vi "Check IP Config.vi"(7 "Retry wait time [ms]":u32=2000, 8 "Error In":errorcluster, 10 "TCP Configuration":T5, 11 "LINX Resource":T1) -> (0 "error out":errorcluster, 2 "TCP Config out":T5, 3 "LINX Resource Out":T1)   [LabVIEW 2019, in "LINXx.lvlib"]
uses:
  LINXx.lvlib
  <vilib>/MakerHub/LINX/Private/Device/Type Defs/TCP Config.ctl
  <vilib>/MakerHub/LINX/Private/Type Defs/LINX Ref.ctl
  <vilib>/MakerHub/LINX/Private/Type Defs/Platform.ctl
  <vilib>/MakerHub/LINX/Private/Type Defs/Interface.ctl
  <vilib>/MakerHub/LINX/Private/Device/Type Defs/LINX Device Config.ctl
  <vilib>/MakerHub/LINX/Private/Device/Type Defs/Channels.ctl
  <vilib>/Utility/error.llb/DialogType.ctl
  Public/Reset Target.ctl
  <vilib>/Utility/error.llb/Error Cluster From Error Code.vi
  <vilib>/ErrorRing/Error Ring.xnode
  <vilib>/MakerHub/LINX/Private/Device/Device.lvlib
  <vilib>/MakerHub/LINX/LMH-LINX.lvlib
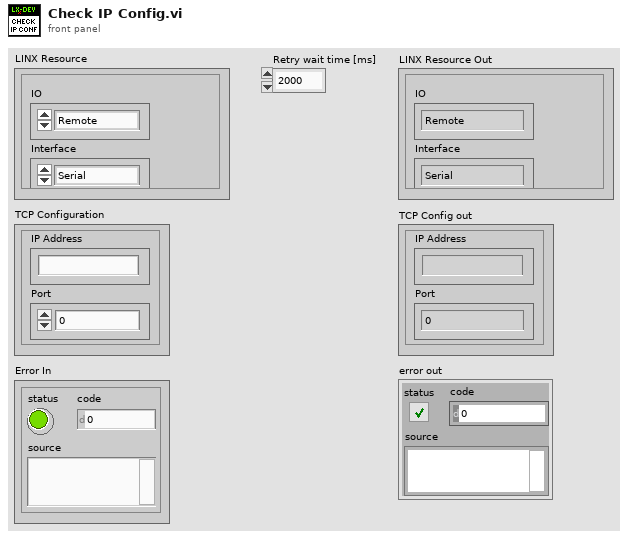
[diagram p1: front panel]
types:
  T1 = typedef "LMH-LINX.lvlib/LINX Ref.ctl" = cluster{"IO":T2, "Interface":T3, "LINX Device Config":T4}
  T2 = typedef "LMH-LINX.lvlib/Platform.ctl" = enum16{"Remote", "Local"}
  T3 = typedef "LMH-LINX.lvlib/Interface.ctl" = enum16{"Serial", "TCP"}
  T4 = typedef "LMH-LINX.lvlib/Device.lvlib/LINX Device Config.ctl" = cluster{"Interface":T3, "COM Port":refnum<visa-resource-name>, "TCP Configuration":T5, "Device Family":u8, "Device ID":u8, "Device Name":string, "TCP Ref":refnum<k5>, "Channels":T6}
  T5 = typedef "LMH-LINX.lvlib/Device.lvlib/TCP Config.ctl" = cluster{"IP Address":string, "Port":u16}
  T6 = typedef "LMH-LINX.lvlib/Channels.ctl" = cluster{"DI":u8[], "DO":u8[], "AI":u8[], "AO":u8[], "PWM":u8[], "QE":u8[], "UART":u8[], "I2C 2":u8[], "SPI":u8[], "CAN":u8[], "Servo":u8[], "AI Ref (V)":dbl, "AI Resolution (Bits)":u8, "AO Ref (V)":dbl, "AO Resolution (Bits)":u8}
  T7 = typedef "DialogType.ctl" = u16
  T8 = typedef "LINXx.lvlib/Reset Target.ctl" = enum16{"None", "Serial", "TCP", "Board"}
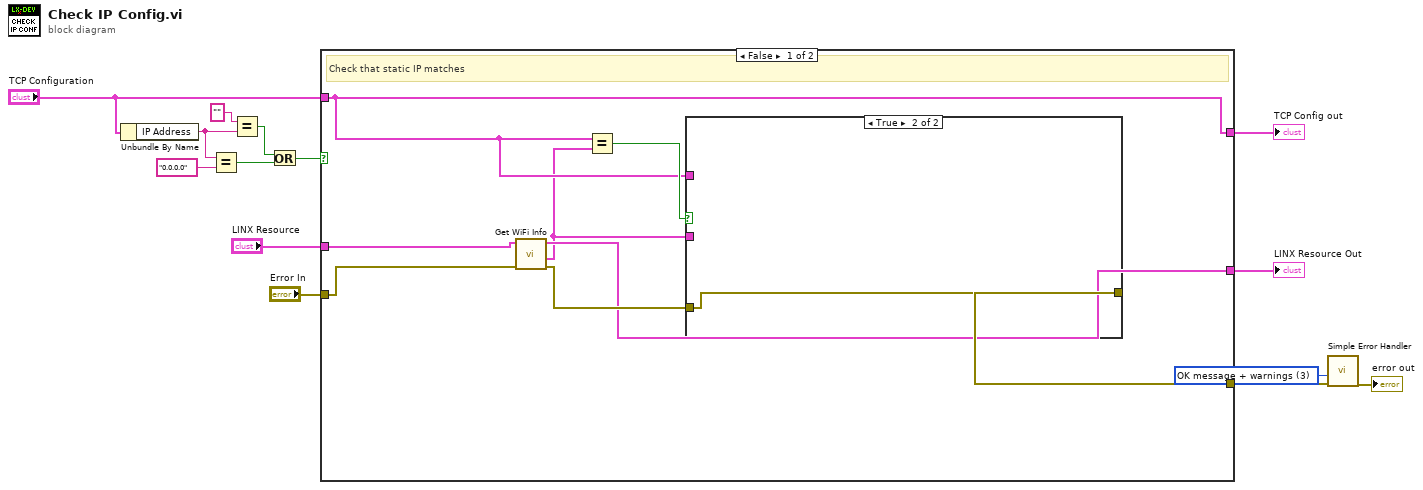
[diagram p0: block diagram]
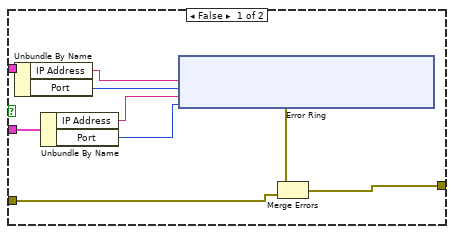
[diagram p2: hidden frame]
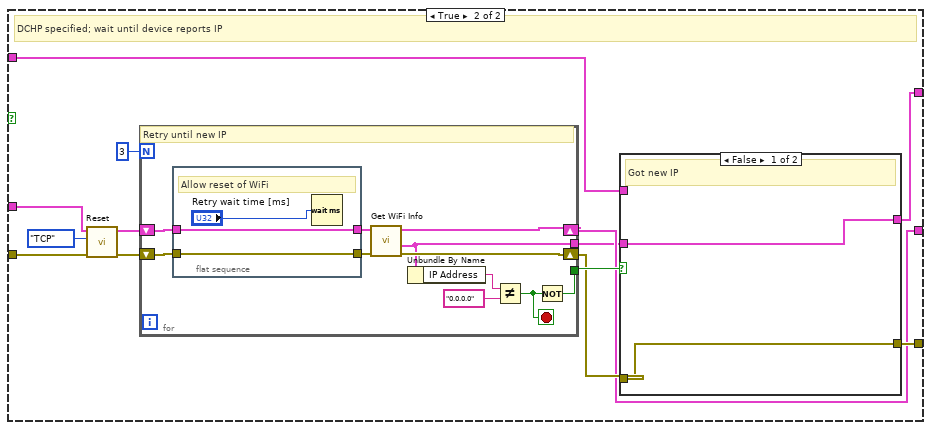
[diagram p3: hidden frame]
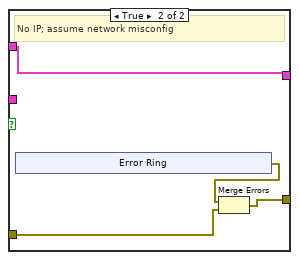
[diagram p4: hidden frame]
diagram:
  w1 = T7 3 items=["no dialog", "OK message", "continue or stop message", "OK message + warnings", "continue/stop + warnings"] ("type of dialog (OK msg:1)")
  n1 = Unbundle By Name("TCP Configuration") -> ("IP Address"=w5:string)
  n2 = Equal?(x=w5, y="0.0.0.0") -> (x = y?=w11:bool)
  n3 = Equal?(x="", y=w5) -> (x = y?=w6:bool)
  n4 = Or(x=w6, y=w11) -> (x .or. y?=w7:bool)
  n5 = case shown="False" w7 {
    tunnel: "Error In" -> [w22 w53]
    tunnel: "LINX Resource" -> [w21 w51]
    tunnel: [w17 w44] -> w8
    tunnel: "TCP Configuration" -> [w16 w47]
    tunnel: [w16 w46] -> w9
    tunnel: [w18 w45] -> w3
    frame False {
      # "Check that static IP matches"
      n6 = call "Get WiFi Info.vi"("Error In"=w22, "LINX Resource"=w21) -> ("Error Out"=w19:errorcluster, "TCP Config"=w15:T5, "LINX Resource Out"=w17:T1)  [unwired: 6 in, 1 out]
      n7 = Equal?(x=w16, y=w15) -> (x = y?=w20:bool)
      n8 = case shown="True" w20 {
        tunnel: w19 -> [w30 w42]
        tunnel: [w29 w42] -> w18
        tunnel: w16 -> [w28 _]
        tunnel: w15 -> [w23 _]
        frame False {
          n9 = Unbundle By Name(w28) -> ("IP Address"=w27:string, "Port"=w26:u16)
          n10 = Unbundle By Name(w23) -> ("IP Address"=w25:string, "Port"=w24:u16)
          n11 = xnode "Error Ring"("parameter 0"=w27, "parameter 1"=w26, "parameter 2"=w25, "parameter 3"=w24) -> ("error out"=w31:errorcluster)
          n12 = Merge Errors(w31, w30) -> (w29:errorcluster)
        }
        frame True {
        }
      }
    }
    frame True {
      # "DCHP specified; wait until device reports IP"
      n13 = call "Reset.vi"("Error In"=w53, "Reset Target"=Reset_Target."TCP", "LINX Resource"=w51) -> ("Error Out"=w52:errorcluster, "LINX Resource out"=w50:T1)  [unwired: 7 in]
      n14 = for {
        N: 3 -> [_]
        shift-right: [w76] -> w44
        shift-left: w50 -> [w72]
        shift-right: [w75] -> w48
        shift-left: w52 -> [w70]
        tunnel: [w73] -> w49
        tunnel: [w68] -> w43
        stop <- w74 stop-if-true
        # "Retry until new IP"
        n15 = flat-sequence {
          tunnel: w72 -> [w79]
          tunnel: [w79] -> w71
          tunnel: w70 -> [w78]
          tunnel: [w78] -> w69
          frame #0 {
            # "Allow reset of WiFi"
            n16 = Wait (ms)(milliseconds to wait="Retry wait time [ms]") -> ()  [unwired: 1 out]
          }
        }
        n17 = call "Get WiFi Info.vi"("Error In"=w69, "LINX Resource"=w71) -> ("Error Out"=w75:errorcluster, "TCP Config"=w68:T5, "LINX Resource Out"=w76:T1)  [unwired: 6 in, 1 out]
        n18 = Unbundle By Name(w68) -> ("IP Address"=w67:string)
        n19 = Not Equal?(x=w67, y="0.0.0.0") -> (x != y?=w74:bool)
        n20 = Not(x=w74) -> (.not. x?=w73:bool)
      }
      n21 = case shown="False" w49 {
        tunnel: w48 -> [w57 w59]
        tunnel: w47 -> [_ w61]
        tunnel: [w56 w61] -> w46
        tunnel: [w57 w58] -> w45
        tunnel: w43 -> [w56 _]
        frame False {
          # "Got new IP"
        }
        frame True {
          # "No IP; assume network misconfig"
          n22 = xnode "Error Ring"() -> ("error out"=w60:errorcluster)
          n23 = Merge Errors(w60, w59) -> (w58:errorcluster)
        }
      }
    }
  }
  "TCP Config out" <- w9
  "LINX Resource Out" <- w8
  n24 = call <vilib>:"Simple Error Handler.vi"("type of dialog (OK msg:1)"=w1, "error in (no error)"=w3) -> ("error out"=→"error out":errorcluster)  [unwired: 3 in, 4 out]
